vi "S4GUI.vi"(7 "Tab ObsEng":enum32{"Obs", "CCD modes", "Eng"}(tab)) -> ()   [LabVIEW 2018] (continued)
                      tunnel: [cluster{u32, u32}[] [{9868950, 9868950}, {9868950, 9868950}] ("Colors [4]") cluster{u32, u32}[] [{9868950, 9868950}, {9868950, 9868950}] ("Colors [4]") cluster{u32, u32}[] [{16318208, 16318208}, {16318208, 16318208}] ("Colors [4]") cluster{u32, u32}[] [{6618880, 6618880}, {6618880, 6618880}] ("Colors [4]") cluster{u32, u32}[] [{16318208, 16318208}, {16318208, 16318208}] ("Colors [4]")] -> w472
                      tunnel: [FALSE ("WPROT Status") FALSE ("WPROT Status") TRUE ("WPROT Status") FALSE ("WPROT Status") TRUE ("WPROT Status")] -> w471
                      frame Default {
                      }
                      frame 0 {
                      }
                      frame 1 {
                      }
                      frame 2 {
                      }
                      frame 3 {
                      }
                    }
                    "WPROT Status" <- w471
                    n230 = property on="WPROT Status" class="Bool (strict)"("Colors [4]"=w472) -> ()  [unwired: 2 in, 2 out]
                  }
                  frame #2 {
                    # "CALW"
                    n231 = Unbundle By Name(w492) -> ("CALW State"=w491:i32)
                    n232 = Unbundle By Name(w490) -> ("CALW posname"=w489:string)
                    n233 = local read "CALW Status"() -> (w485:bool)
                    n234 = case shown="3" w491 {
                      tunnel: [cluster{u32, u32}[] [{9868950, 9868950}, {9868950, 9868950}] ("Colors [4]") cluster{u32, u32}[] [{9868950, 9868950}, {9868950, 9868950}] ("Colors [4]") cluster{u32, u32}[] [{16318208, 16318208}, {16318208, 16318208}] ("Colors [4]") cluster{u32, u32}[] [{6618880, 6618880}, {6618880, 6618880}] ("Colors [4]") w512] -> w486
                      tunnel: [FALSE ("WPROT Status") FALSE ("WPROT Status") TRUE ("WPROT Status") FALSE ("WPROT Status") w514] -> w488
                      tunnel: w489 -> [_ _ _ w503 _]
                      tunnel: ["" "" "" w502 ""] -> w487
                      tunnel: w485 -> [_ _ _ _ w513]
                      frame Default {
                      }
                      frame 0 {
                      }
                      frame 1 {
                      }
                      frame 2 {
                        n235 = case shown="\"SHUTTER\"" w503 {
                          tunnel: ["" "DEPOL" "POL" "OFF" "PIN" "SHT"] -> w502
                          frame Default {
                          }
                          frame "DEPOLARIZER" {
                          }
                          frame "POLARIZER" {
                          }
                          frame "OFF" {
                          }
                          frame "PINHOLE" {
                          }
                          frame "SHUTTER" {
                          }
                        }
                      }
                      frame 3 {
                        n236 = case shown="False" w513 {
                          tunnel: [cluster{u32, u32}[] [{7563008, 7563008}, {7563008, 7563008}] ("Colors [4]") cluster{u32, u32}[] [{16318208, 16318208}, {16318208, 16318208}] ("Colors [4]")] -> w512
                          frame False {
                          }
                          frame True {
                          }
                        }
                        n237 = Not(x=w513) -> (.not. x?=w514:bool)
                      }
                    }
                    "CALW Status" <- w488
                    "PCS" <- w488
                    n238 = property on="CALW Status" class="Bool (strict)"("Colors [4]"=w486) -> ()  [unwired: 2 in, 2 out]
                    n239 = property on="PCS" class="Bool (strict)"("Colors [4]"=w486, "BoolText.Text"=w487) -> ()  [unwired: 2 in, 2 out]
                  }
                  frame #3 {
                    # "ASEL"
                    n240 = Unbundle By Name(w526) -> ("ASEL State"=w525:i32)
                    n241 = Unbundle By Name(w522) -> ("ASEL posname"=w519:string)
                    n242 = local read "ASEL Status"() -> (w520:bool)
                    n243 = case shown="Default" w519 {
                      selector: w519 -> [w527 _ _]
                      tunnel: [w527 "OFF" ("y") "ON" ("y")] -> w518
                      frame Default {
                      }
                      frame "OFF" {
                      }
                      frame "ON" {
                      }
                    }
                    n244 = case shown="3" w525 {
                      tunnel: [cluster{u32, u32}[] [{9868950, 9868950}, {9868950, 9868950}] ("Colors [4]") cluster{u32, u32}[] [{9868950, 9868950}, {9868950, 9868950}] ("Colors [4]") cluster{u32, u32}[] [{16318208, 16318208}, {16318208, 16318208}] ("Colors [4]") cluster{u32, u32}[] [{6618880, 6618880}, {6618880, 6618880}] ("Colors [4]") w545] -> w523
                      tunnel: [FALSE ("WPROT Status") FALSE ("WPROT Status") TRUE FALSE ("WPROT Status") w544] -> w524
                      tunnel: w518 -> [_ _ _ w540 _]
                      tunnel: ["" ("y") "" ("y") "" ("y") w540 "" ("y")] -> w521
                      tunnel: w520 -> [_ _ _ _ w542]
                      frame Default {
                      }
                      frame 0 {
                      }
                      frame 1 {
                      }
                      frame 2 {
                      }
                      frame 3 {
                        n245 = case shown="True" w542 {
                          tunnel: [cluster{u32, u32}[] [{7563008, 7563008}, {7563008, 7563008}] ("Colors [4]") cluster{u32, u32}[] [{16318208, 16318208}, {16318208, 16318208}] ("Colors [4]")] -> w545
                          frame False {
                          }
                          frame True {
                          }
                        }
                        n246 = Not(x=w542) -> (.not. x?=w544:bool)
                      }
                    }
                    "ASEL Status" <- w524
                    "Analyzer" <- w524
                    n247 = property on="Analyzer" class="Bool (strict)"("Colors [4]"=w523, "BoolText.Text"=w521) -> ()  [unwired: 2 in, 2 out]
                    n248 = property on="ASEL Status" class="Bool (strict)"("Colors [4]"=w523) -> ()  [unwired: 2 in, 2 out]
                  }
                  frame #4 {
                    # "GMIR"
                    n249 = Unbundle By Name(w551) -> ("GMIR State"=w550:i32)
                    n250 = case shown="0" w550 {
                      tunnel: [cluster{u32, u32}[] [{9868950, 9868950}, {9868950, 9868950}] ("Colors [4]") cluster{u32, u32}[] [{9868950, 9868950}, {9868950, 9868950}] ("Colors [4]") cluster{u32, u32}[] [{16318208, 16318208}, {16318208, 16318208}] ("Colors [4]") cluster{u32, u32}[] [{6618880, 6618880}, {6618880, 6618880}] ("Colors [4]") cluster{u32, u32}[] [{16318208, 16318208}, {16318208, 16318208}] ("Colors [4]")] -> w549
                      tunnel: [FALSE ("WPROT Status") FALSE ("WPROT Status") TRUE ("WPROT Status") FALSE ("WPROT Status") TRUE ("WPROT Status")] -> w548
                      frame Default {
                      }
                      frame 0 {
                      }
                      frame 1 {
                      }
                      frame 2 {
                      }
                      frame 3 {
                      }
                    }
                    "GMIR Status" <- w548
                    n251 = property on="GMIR Status" class="Bool (strict)"("Colors [4]"=w549) -> ()  [unwired: 2 in, 2 out]
                  }
                  frame #5 {
                    # "GFOC"
                    n252 = Unbundle By Name(w565) -> ("GFOC State"=w564:i32)
                    n253 = case shown="2" w564 {
                      tunnel: [cluster{u32, u32}[] [{9868950, 9868950}, {9868950, 9868950}] ("Colors [4]") cluster{u32, u32}[] [{9868950, 9868950}, {9868950, 9868950}] ("Colors [4]") cluster{u32, u32}[] [{16318208, 16318208}, {16318208, 16318208}] ("Colors [4]") cluster{u32, u32}[] [{6618880, 6618880}, {6618880, 6618880}] ("Colors [4]") cluster{u32, u32}[] [{16318208, 16318208}, {16318208, 16318208}] ("Colors [4]")] -> w563
                      tunnel: [FALSE ("WPROT Status") FALSE ("WPROT Status") TRUE ("WPROT Status") FALSE ("WPROT Status") TRUE ("WPROT Status")] -> w562
                      frame Default {
                      }
                      frame 0 {
                      }
                      frame 1 {
                      }
                      frame 2 {
                      }
                      frame 3 {
                      }
                    }
                    "GFOC Status" <- w562
                    n254 = property on="GFOC Status" class="Bool (strict)"("Colors [4]"=w563) -> ()  [unwired: 2 in, 2 out]
                  }
                }
              }
              frame #7 {
                n255 = Unbundle By Name(w578) -> ("Instrument Pos Names"=w577:T20)
                n256 = stacked-sequence {
                  tunnel: w577 -> [w580 w597 w622 w648]
                  tunnel: [_ _ _ w649] -> w576
                  frame #0 {
                    n257 = Unbundle By Name(w580) -> ("WPSEL posname"=w579:string)
                    n258 = case shown="\"L/2\", \"L/4\", \"OFF\"" w579 {
                      selector: w579 -> [_ w581]
                      frame "False", Default {
                      }
                      frame "L/2", "L/4", "OFF" {
                        n259 = First Call?() -> (First Call?: T/F=w582:bool)
                        n260 = case shown="True" w582 {
                          tunnel: w581 -> [_ w583]
                          frame False {
                          }
                          frame True {
                            n261 = case shown="\"L/2\"" w583 {
                              frame "False", Default {
                              }
                              frame "L/2" {
                                w584 = u16 1 items=["OFF", "Lambda/2", "Lambda/4"] ("Lambda Selector")
                                n262 = property on="Lambda Selector" class="Ring (strict)"(error in=errorcluster {"status"=FALSE, "code"=0, "source"=""} ("error in (no error)"), "Value"=w584) -> (error out=w586:errorcluster)  [unwired: 1 in, 1 out]
                                n263 = property on="Lambda Selector" class="Ring (strict)"(error in=w586, "RingText.Text"="Lambda/2" ("Boolean Text.Text")) -> ()  [unwired: 1 in, 2 out]
                              }
                              frame "L/4" {
                                w588 = u16 2 items=["OFF", "Lambda/2", "Lambda/4"] ("Lambda Selector")
                                n264 = property on="Lambda Selector" class="Ring (strict)"(error in=errorcluster {"status"=FALSE, "code"=0, "source"=""} ("error in (no error)"), "Value"=w588) -> (error out=w590:errorcluster)  [unwired: 1 in, 1 out]
                                n265 = property on="Lambda Selector" class="Ring (strict)"(error in=w590, "RingText.Text"="Lambda/4" ("Boolean Text.Text")) -> ()  [unwired: 1 in, 2 out]
                              }
                              frame "OFF" {
                                w592 = u16 0 items=["OFF", "Lambda/2", "Lambda/4"] ("Lambda Selector")
                                n266 = property on="Lambda Selector" class="Ring (strict)"(error in=errorcluster {"status"=FALSE, "code"=0, "source"=""} ("error in (no error)"), "Value"=w592) -> (error out=w594:errorcluster)  [unwired: 1 in, 1 out]
                                n267 = property on="Lambda Selector" class="Ring (strict)"(error in=w594, "RingText.Text"="OFF" ("Boolean Text.Text")) -> ()  [unwired: 1 in, 2 out]
                              }
                            }
                          }
                        }
                      }
                    }
                  }
                  frame #1 {
                    n268 = Unbundle By Name(w597) -> ("CALW posname"=w596:string)
                    n269 = case shown="\"DEPOLARIZER\", \"OFF\", \"PINHOLE\", \"POLARIZER\", \"SHUTTER\"" w596 {
                      selector: w596 -> [_ w598]
                      frame "False", Default {
                      }
                      frame "DEPOLARIZER", "OFF", "PINHOLE", "POLARIZER", "SHUTTER" {
                        n270 = First Call?() -> (First Call?: T/F=w599:bool)
                        n271 = case shown="True" w599 {
                          tunnel: w598 -> [_ w600]
                          frame False {
                          }
                          frame True {
                            n272 = case shown="\"OFF\"" w600 {
                              frame "False", Default {
                              }
                              frame "POLARIZER" {
                                w601 = u16 1 items=["OFF", "POLARIZER", "PINHOLE", "SHUTTER", "DEPOLARIZER"] ("Calibrator Selector")
                                n273 = property on="Calibrator Selector" class="Ring (strict)"(error in=errorcluster {"status"=FALSE, "code"=0, "source"=""} ("error in (no error)"), "Value"=w601) -> (error out=w603:errorcluster)  [unwired: 1 in, 1 out]
                                n274 = property on="Calibrator Selector" class="Ring (strict)"(error in=w603, "RingText.Text"="POLARIZER" ("Boolean Text.Text")) -> ()  [unwired: 1 in, 2 out]
                              }
                              frame "DEPOLARIZER" {
                                w605 = u16 4 items=["OFF", "POLARIZER", "PINHOLE", "SHUTTER", "DEPOLARIZER"] ("Calibrator Selector")
                                n275 = property on="Calibrator Selector" class="Ring (strict)"(error in=errorcluster {"status"=FALSE, "code"=0, "source"=""} ("error in (no error)"), "Value"=w605) -> (error out=w607:errorcluster)  [unwired: 1 in, 1 out]
                                n276 = property on="Calibrator Selector" class="Ring (strict)"(error in=w607, "RingText.Text"="DEPOLARIZER" ("Boolean Text.Text")) -> ()  [unwired: 1 in, 2 out]
                              }
                              frame "PINHOLE" {
                                w609 = u16 2 items=["OFF", "POLARIZER", "PINHOLE", "SHUTTER", "DEPOLARIZER"] ("Calibrator Selector")
                                n277 = property on="Calibrator Selector" class="Ring (strict)"(error in=errorcluster {"status"=FALSE, "code"=0, "source"=""} ("error in (no error)"), "Value"=w609) -> (error out=w611:errorcluster)  [unwired: 1 in, 1 out]
                                n278 = property on="Calibrator Selector" class="Ring (strict)"(error in=w611, "RingText.Text"="PINHOLE" ("Boolean Text.Text")) -> ()  [unwired: 1 in, 2 out]
                              }
                              frame "SHUTTER" {
                                w613 = u16 3 items=["OFF", "POLARIZER", "PINHOLE", "SHUTTER", "DEPOLARIZER"] ("Calibrator Selector")
                                n279 = property on="Calibrator Selector" class="Ring (strict)"(error in=errorcluster {"status"=FALSE, "code"=0, "source"=""} ("error in (no error)"), "Value"=w613) -> (error out=w615:errorcluster)  [unwired: 1 in, 1 out]
                                n280 = property on="Calibrator Selector" class="Ring (strict)"(error in=w615, "RingText.Text"="SHUTTER" ("Boolean Text.Text")) -> ()  [unwired: 1 in, 2 out]
                              }
                              frame "OFF" {
                                w617 = u16 0 items=["OFF", "POLARIZER", "PINHOLE", "SHUTTER", "DEPOLARIZER"] ("Calibrator Selector")
                                n281 = property on="Calibrator Selector" class="Ring (strict)"(error in=errorcluster {"status"=FALSE, "code"=0, "source"=""} ("error in (no error)"), "Value"=w617) -> (error out=w619:errorcluster)  [unwired: 1 in, 1 out]
                                n282 = property on="Calibrator Selector" class="Ring (strict)"(error in=w619, "RingText.Text"="OFF" ("Boolean Text.Text")) -> ()  [unwired: 1 in, 2 out]
                              }
                            }
                          }
                        }
                      }
                    }
                  }
                  frame #2 {
                    n283 = Unbundle By Name(w622) -> ("WPROT posname"=w621:string)
                    "Name" <- w621
                    n284 = stacked-sequence {
                      tunnel: w621 -> [_ w624]
                      frame #0 {
                        w623 = FALSE
                        "ledP0" <- w623
                        "ledP1" <- w623
                        "ledP2" <- w623
                        "ledP3" <- w623
                        "ledP4" <- w623
                        "ledP5" <- w623
                        "ledP6" <- w623
                        "ledP7" <- w623
                        "ledP8" <- w623
                        "ledP9" <- w623
                        "ledP10" <- w623
                        "ledP11" <- w623
                        "ledP12" <- w623
                        "ledP13" <- w623
                        "ledP14" <- w623
                        "ledP15" <- w623
                      }
                      frame #1 {
                        n285 = case shown="\"WP3\"" w624 {
                          frame Default {
                          }
                          frame "WP1" {
                            n286 = local write "ledP0"(TRUE ("ledP0")) -> ()
                          }
                          frame "WP2" {
                            n287 = local write "ledP1"(TRUE ("ledP0")) -> ()
                          }
                          frame "WP3" {
                            n288 = local write "ledP2"(TRUE ("ledP0")) -> ()
                          }
                          frame "WP4" {
                            n289 = local write "ledP3"(TRUE ("ledP0")) -> ()
                          }
                          frame "WP5" {
                            n290 = local write "ledP4"(TRUE ("ledP0")) -> ()
                          }
                          frame "WP6" {
                            n291 = local write "ledP5"(TRUE ("ledP0")) -> ()
                          }
                          frame "WP7" {
                            n292 = local write "ledP6"(TRUE ("ledP0")) -> ()
                          }
                          frame "WP8" {
                            n293 = local write "ledP7"(TRUE ("ledP0")) -> ()
                          }
                          frame "WP9" {
                            n294 = local write "ledP8"(TRUE ("ledP0")) -> ()
                          }
                          frame "WP10" {
                            n295 = local write "ledP9"(TRUE ("ledP0")) -> ()
                          }
                          frame "WP11" {
                            n296 = local write "ledP10"(TRUE ("ledP0")) -> ()
                          }
                          frame "WP12" {
                            n297 = local write "ledP11"(TRUE ("ledP0")) -> ()
                          }
                          frame "WP13" {
                            n298 = local write "ledP12"(TRUE ("ledP0")) -> ()
                          }
                          frame "WP14" {
                            n299 = local write "ledP13"(TRUE ("ledP0")) -> ()
                          }
                          frame "WP15" {
                            n300 = local write "ledP14"(TRUE ("ledP0")) -> ()
                          }
                          frame "WP16" {
                            n301 = local write "ledP15"(TRUE ("ledP0")) -> ()
                          }
                        }
                      }
                    }
                  }
                  frame #3 {
                    w652 = "OFF" ("Boolean Text.Text")
                    # "Polarimetria:   ASEL = ON  &   (WPSEL =L/2 or L/4)\n\nFotometria:    ASEL=OFF & WPSEL = OFF & CALW = OFF"
                    n302 = Unbundle By Name(w648) -> ("ASEL posname"=w643:string, "WPSEL posname"=w645:string, "CALW posname"=w644:string)
                    n303 = Unbundle By Name(w648) -> ("WPSEL posname"=w655:string, "CALW posname"=w656:string, "ASEL posname"=w650:string)
                    n304 = Equal?(x=w643, y="ON" ("Boolean Text.Text")) -> (x = y?=w646:bool)
                    n305 = case shown="True" w646 {
                      tunnel: w645 -> [w665 w674]
                      tunnel: w644 -> [w664 w668]
                      tunnel: w643 -> [w661 _]
                      tunnel: [FALSE ("Polarimetric Mode") w669] -> w642
                      tunnel: [w657 FALSE ("Photometric Mode")] -> w641
                      frame False {
                        w660 = "OFF" ("Boolean Text.Text")
                        n306 = Equal?(x=w661, y=w660) -> (x = y?=w659:bool)
                        n307 = Equal?(x=w664, y=w660) -> (x = y?=w662:bool)
                        n308 = Equal?(x=w665, y=w660) -> (x = y?=w663:bool)
                        n309 = Compound Arithmetic op=AND(w659, w663, w662) -> (w657:bool)
                      }
                      frame True {
                        n310 = Equal?(x="L/2" ("Boolean Text.Text"), y=w674) -> (x = y?=w675:bool)
                        n311 = Equal?(x="L/4" ("Boolean Text.Text"), y=w674) -> (x = y?=w672:bool)
                        n312 = Not Equal?(x="SHUTTER", y=w668) -> (x != y?=w666:bool)
                        n313 = Or(x=w675, y=w672) -> (x .or. y?=w670:bool)
                        n314 = And(x=w670, y=w666) -> (x .and. y?=w669:bool)
                      }
                    }
                    "Polarimetric Mode" <- w642
                    "Photometric Mode" <- w641
                    n315 = Equal?(x=w652, y=w655) -> (x = y?=w653:bool)
                    n316 = Equal?(x=w652, y=w656) -> (x = y?=w654:bool)
                    n317 = Equal?(x=w652, y=w650) -> (x = y?=w651:bool)
                    n318 = Compound Arithmetic op=AND(w653, w654, w651) -> (invert w649:bool)
                  }
                }
              }
              frame #8 {
                n319 = Unbundle By Name(w681) -> ("ChannelA_Status"=w680:T21, "ChannelB_Status"=w679:T21, "ChannelC_Status"=w677:T21, "ChannelD_Status"=w678:T21)
                n320 = stacked-sequence {
                  tunnel: w680 -> [w769 w825 w877 w954 _ _ _]
                  tunnel: w679 -> [w768 w823 w876 _ w975 _ _]
                  tunnel: w678 -> [w766 w820 w874 _ _ _ w1017]
                  tunnel: w677 -> [w767 w821 w875 _ _ w996 _]
                  frame #0 {
                    n321 = Unbundle By Name(w766) -> ("connection"=w746:bool, "FT"=w727:bool, "Current exp"=w704:dbl, "Cooler ON/OFF"=w760:i16, "Currently temperature"=w757:i16, "Temperature Status"=w754:string, "target  temp"=w689:i16)
                    "Exposure Time ch4" <- w704
                    n322 = Unbundle By Name(w768) -> ("connection"=w748:bool, "FT"=w731:bool, "Current exp"=w715:dbl, "Cooler ON/OFF"=w762:i16, "Currently temperature"=w759:i16, "Temperature Status"=w756:string, "target  temp"=w693:i16)
                    "Exposure Time ch2" <- w715
                    n323 = Unbundle By Name(w769) -> ("connection"=w749:bool, "FT"=w732:bool, "Current exp"=w724:dbl, "Cooler ON/OFF"=w765:i16, "Currently temperature"=w763:i16, "Temperature Status"=w764:string, "target  temp"=w701:i16)
                    "Exposure Time ch1" <- w724
                    n324 = Unbundle By Name(w767) -> ("connection"=w747:bool, "FT"=w729:bool, "Current exp"=w705:dbl, "Cooler ON/OFF"=w761:i16, "Currently temperature"=w758:i16, "Temperature Status"=w755:string, "target  temp"=w690:i16)
                    "Exposure Time ch3" <- w705
                    n325 = Number To Decimal String(number=w689) -> (decimal integer string=→"Target Temp 4":string)  [unwired: 1 in]
                    n326 = Number To Decimal String(number=w690) -> (decimal integer string=→"Target Temp 3":string)  [unwired: 1 in]
                    n327 = Number To Decimal String(number=w693) -> (decimal integer string=→"Target Temp 2":string)  [unwired: 1 in]
                    n328 = Not Equal To 0?(x=w760) -> (x != 0?=w751:bool)
                    n329 = First Call?() -> (First Call?: T/F=w743:bool)
                    n330 = First Call?() -> (First Call?: T/F=w745:bool)
                    n331 = First Call?() -> (First Call?: T/F=w742:bool)
                    n332 = Not Equal To 0?(x=w761) -> (x != 0?=w750:bool)
                    n333 = First Call?() -> (First Call?: T/F=w744:bool)
                    n334 = Number To Decimal String(number=w701) -> (decimal integer string=→"Target Temp 1":string)  [unwired: 1 in]
                    n335 = Number To Fractional String(use system decimal point (T)=FALSE, number=w724, precision (6)=i16 2) -> (F-format string=w721:string)  [unwired: 1 in]
                    n336 = case shown="True" w743 {
                      tunnel: w690 -> [_ w771]
                      frame False {
                      }
                      frame True {
                        n337 = property on="Target Temp 3" class="DigNum (strict)"("Value"=w771) -> ()  [unwired: 2 in, 2 out]
                      }
                    }
                    n338 = case shown="True" w745 {
                      tunnel: w701 -> [_ w773]
                      frame False {
                      }
                      frame True {
                        n339 = property on="Target Temp 1" class="DigNum (strict)"("Value"=w773) -> ()  [unwired: 2 in, 2 out]
                      }
                    }
                    n340 = Number To Fractional String(use system decimal point (T)=FALSE, number=w715, precision (6)=i16 2) -> (F-format string=w716:string)  [unwired: 1 in]
                    n341 = case shown="True" w742 {
                      tunnel: w689 -> [_ w770]
                      frame False {
                      }
                      frame True {
                        n342 = property on="Target Temp 4" class="DigNum (strict)"("Value"=w770) -> ()  [unwired: 2 in, 2 out]
                      }
                    }
                    n343 = Concatenate Strings("Exposure Time ", w721) -> (w720:string)
                    n344 = Number To Fractional String(use system decimal point (T)=FALSE, number=w705, precision (6)=i16 2) -> (F-format string=w706:string)  [unwired: 1 in]
                    n345 = Number To Fractional String(use system decimal point (T)=FALSE, number=w704, precision (6)=i16 2) -> (F-format string=w710:string)  [unwired: 1 in]
                    n346 = Concatenate Strings("Exposure Time ", w716) -> (w714:string)
                    n347 = case shown="True" w744 {
                      tunnel: w693 -> [_ w772]
                      frame False {
                      }
                      frame True {
                        n348 = property on="Target Temp 2" class="DigNum (strict)"("Value"=w772) -> ()  [unwired: 2 in, 2 out]
                      }
                    }
                    n349 = Concatenate Strings("Exposure Time ", w706) -> (w702:string)
                    n350 = Concatenate Strings("Exposure Time ", w710) -> (w703:string)
                    n351 = property on="Exposure Time ch1" class="Slide (strict)"("Caption.Text"=w720) -> ()  [unwired: 2 in, 2 out]
                    n352 = property on="Exposure Time ch2" class="Slide (strict)"("Caption.Text"=w714) -> ()  [unwired: 2 in, 2 out]
                    n353 = property on="Exposure Time ch3" class="Slide (strict)"("Caption.Text"=w702) -> ()  [unwired: 2 in, 2 out]
                    n354 = property on="Exposure Time ch4" class="Slide (strict)"("Caption.Text"=w703) -> ()  [unwired: 2 in, 2 out]
                    n355 = Not Equal To 0?(x=w765) -> (x != 0?=w752:bool)
                    n356 = Not Equal To 0?(x=w762) -> (x != 0?=w753:bool)
                    n357 = case shown="False" w749 {
                      tunnel: w764 -> [_ w803]
                      tunnel: w763 -> [_ w804]
                      tunnel: w752 -> [_ w805]
                      tunnel: [FALSE w805] -> w741
                      tunnel: [i16 0 ("Currently temperature") w804] -> w698
                      tunnel: ["" ("Temperature Status") w803] -> w740
                      tunnel: [FALSE w802] -> w733
                      tunnel: w732 -> [_ w802]
                      frame False {
                      }
                      frame True {
                      }
                    }
                    "Cooler status 1" <- w741
                    "Curr Temp 1" <- w698
                    "Temp Status 1" <- w740
                    "Panel Temp" <- w698
                    "Panel cooler 1" <- w741
                    "FT1" <- w733
                    n358 = case shown="False" w748 {
                      tunnel: w759 -> [_ w796]
                      tunnel: w756 -> [_ w795]
                      tunnel: w753 -> [_ w797]
                      tunnel: [FALSE w797] -> w739
                      tunnel: [i16 0 ("Currently temperature") w796] -> w694
                      tunnel: ["" ("Temperature Status") w795] -> w738
                      tunnel: w731 -> [_ w794]
                      tunnel: [FALSE ("FT") w794] -> w730
                      frame False {
                      }
                      frame True {
                      }
                    }
                    "Panel Temp 2" <- w694
                    "Curr Temp 2" <- w694
                    "Cooler status 2" <- w739
                    "Panel cooler 2" <- w739
                    "Temp Status 2" <- w738
                    "FT2" <- w730
                    n359 = case shown="True" w746 {
                      tunnel: w757 -> [_ w780]
                      tunnel: w754 -> [_ w779]
                      tunnel: w751 -> [_ w781]
                      tunnel: [FALSE w781] -> w735
                      tunnel: [i16 0 ("Currently temperature") w780] -> w682
                      tunnel: ["" ("Temperature Status") w779] -> w734
                      tunnel: w727 -> [_ w778]
                      tunnel: [FALSE ("FT") w778] -> w726
                      frame False {
                      }
                      frame True {
                      }
                    }
                    "Cooler status 4" <- w735
                    "Panel Temp 4" <- w682
                    "Curr Temp 4" <- w682
                    "Temp Status 4" <- w734
                    "Panel cooler 4" <- w735
                    "FT4" <- w726
                    n360 = case shown="True" w747 {
                      tunnel: w758 -> [_ w788]
                      tunnel: w755 -> [_ w787]
                      tunnel: w750 -> [_ w789]
                      tunnel: [FALSE w789] -> w737
                      tunnel: [i16 0 ("Currently temperature") w788] -> w683
                      tunnel: ["" ("Temperature Status") w787] -> w736
                      tunnel: w729 -> [_ w786]
                      tunnel: [FALSE ("FT") w786] -> w728
                      frame False {
                      }
                      frame True {
                      }
                    }
                    "Cooler status 3" <- w737
                    "Panel Temp 3" <- w683
                    "Curr Temp 3" <- w683
                    "Temp Status 3" <- w736
                    "Panel cooler 3" <- w737
                    "FT3" <- w728
                    n361 = Number To Decimal String(number=w694) -> (decimal integer string=w695:string)  [unwired: 1 in]
                    n362 = Number To Decimal String(number=w698) -> (decimal integer string=w699:string)  [unwired: 1 in]
                    n363 = property on="Panel cooler 2" class="Bool (strict)"("BoolText.Text"=w695, "BoolText.Justify"=enum16{"Left", "Center", "Right"}."Right" ("Boolean Text.Justification")) -> ()  [unwired: 2 in, 2 out]
                    n364 = property on="Panel cooler 1" class="Bool (strict)"("BoolText.Text"=w699, "BoolText.Justify"=enum16{"Left", "Center", "Right"}."Right" ("Boolean Text.Justification")) -> ()  [unwired: 2 in, 2 out]
                    n365 = Number To Decimal String(number=w683) -> (decimal integer string=w687:string)  [unwired: 1 in]
                    n366 = Number To Decimal String(number=w682) -> (decimal integer string=w684:string)  [unwired: 1 in]
                    n367 = property on="Panel cooler 3" class="Bool (strict)"("BoolText.Text"=w687, "BoolText.Justify"=enum16{"Left", "Center", "Right"}."Right" ("Boolean Text.Justification")) -> ()  [unwired: 2 in, 2 out]
                    n368 = property on="Panel cooler 4" class="Bool (strict)"("BoolText.Text"=w684, "BoolText.Justify"=enum16{"Left", "Center", "Right"}."Right" ("Boolean Text.Justification")) -> ()  [unwired: 2 in, 2 out]
                  }
                  frame #1 {
                    n369 = Unbundle By Name(w820) -> ("LastFileImage"=→"Last Image ch4":string, "Temperature Status"=w808:string)
                    n370 = Unbundle By Name(w821) -> ("LastFileImage"=→"Last Image ch3":string, "Temperature Status"=w809:string)
                    n371 = Unbundle By Name(w823) -> ("LastFileImage"=→"Last Image ch2":string, "Temperature Status"=w812:string)
                    n372 = Unbundle By Name(w825) -> ("LastFileImage"=→"Last Image ch1":string, "Temperature Status"=w817:string)
                    n373 = case shown="\"TEMPERATURE_NOT_REACHED\"" w817 {
                      tunnel: [cluster{u32, u32}[] [{6124107, 6124107}, {6124107, 6124107}] ("Colors [4]") cluster{u32, u32}[] [{6618880, 6618880}, {6618880, 6618880}] ("Colors [4]") cluster{u32, u32}[] [{16318208, 16318208}, {16318208, 16318208}] ("Colors [4]") cluster{u32, u32}[] [{8554752, 8554752}, {8554752, 8554752}] ("Colors [4]")] -> w816
                      tunnel: [FALSE FALSE FALSE TRUE] -> w815
                      frame Default {
                      }
                      frame "TEMPERATURE_STABILIZED" {
                      }
                      frame "TEMPERATURE_NOT_STABILIZED" {
                      }
                      frame "TEMPERATURE_NOT_REACHED" {
                      }
                    }
                    n374 = case shown="\"TEMPERATURE_NOT_REACHED\"" w812 {
                      tunnel: [cluster{u32, u32}[] [{6124107, 6124107}, {6124107, 6124107}] ("Colors [4]") cluster{u32, u32}[] [{6618880, 6618880}, {6618880, 6618880}] ("Colors [4]") cluster{u32, u32}[] [{16318208, 16318208}, {16318208, 16318208}] ("Colors [4]") cluster{u32, u32}[] [{8554752, 8554752}, {8554752, 8554752}] ("Colors [4]")] -> w814
                      tunnel: [FALSE FALSE FALSE TRUE] -> w813
                      frame Default {
                      }
                      frame "TEMPERATURE_STABILIZED" {
                      }
                      frame "TEMPERATURE_NOT_STABILIZED" {
                      }
                      frame "TEMPERATURE_NOT_REACHED" {
                      }
                    }
                    n375 = case shown="\"TEMPERATURE_NOT_REACHED\"" w809 {
                      tunnel: [cluster{u32, u32}[] [{6124107, 6124107}, {6124107, 6124107}] ("Colors [4]") cluster{u32, u32}[] [{6618880, 6618880}, {6618880, 6618880}] ("Colors [4]") cluster{u32, u32}[] [{16318208, 16318208}, {16318208, 16318208}] ("Colors [4]") cluster{u32, u32}[] [{8554752, 8554752}, {8554752, 8554752}] ("Colors [4]")] -> w811
                      tunnel: [FALSE FALSE FALSE TRUE] -> w810
                      frame Default {
                      }
                      frame "TEMPERATURE_STABILIZED" {
                      }
                      frame "TEMPERATURE_NOT_STABILIZED" {
                      }
                      frame "TEMPERATURE_NOT_REACHED" {
                      }
                    }
                    n376 = case shown="\"TEMPERATURE_NOT_REACHED\"" w808 {
                      tunnel: [cluster{u32, u32}[] [{6124107, 6124107}, {6124107, 6124107}] ("Colors [4]") cluster{u32, u32}[] [{6618880, 6618880}, {6618880, 6618880}] ("Colors [4]") cluster{u32, u32}[] [{16318208, 16318208}, {16318208, 16318208}] ("Colors [4]") cluster{u32, u32}[] [{8554752, 8554752}, {8554752, 8554752}] ("Colors [4]")] -> w807
                      tunnel: [FALSE FALSE FALSE TRUE] -> w806
                      frame Default {
                      }
                      frame "TEMPERATURE_STABILIZED" {
                      }
                      frame "TEMPERATURE_NOT_STABILIZED" {
                      }
                      frame "TEMPERATURE_NOT_REACHED" {
                      }
                    }
                    n377 = property on="Cooler status 1" class="Bool (strict)"("Colors [4]"=w816, "Blinking"=w815) -> ()  [unwired: 2 in, 2 out]
                    n378 = property on="Panel cooler 1" class="Bool (strict)"("Colors [4]"=w816, "Blinking"=w815) -> ()  [unwired: 2 in, 2 out]
                    n379 = property on="Cooler status 4" class="Bool (strict)"("Colors [4]"=w807, "Blinking"=w806) -> ()  [unwired: 2 in, 2 out]
                    n380 = property on="Cooler status 3" class="Bool (strict)"("Colors [4]"=w811, "Blinking"=w810) -> ()  [unwired: 2 in, 2 out]
                    n381 = property on="Panel cooler 4" class="Bool (strict)"("Colors [4]"=w807, "Blinking"=w806) -> ()  [unwired: 2 in, 2 out]
                    n382 = property on="Cooler status 2" class="Bool (strict)"("Colors [4]"=w814, "Blinking"=w813) -> ()  [unwired: 2 in, 2 out]
                    n383 = property on="Panel cooler 3" class="Bool (strict)"("Colors [4]"=w811, "Blinking"=w810) -> ()  [unwired: 2 in, 2 out]
                    n384 = property on="Panel cooler 2" class="Bool (strict)"("Colors [4]"=w814, "Blinking"=w813) -> ()  [unwired: 2 in, 2 out]
                  }
                  frame #2 {
                    n385 = Unbundle By Name(w876) -> ("CamStatus"=w869:string, "connection"=w868:bool)
                    n386 = Unbundle By Name(w875) -> ("CamStatus"=w865:string, "connection"=w864:bool)
                    n387 = Unbundle By Name(w874) -> ("CamStatus"=w861:string, "connection"=w860:bool)
                    n388 = Unbundle By Name(w877) -> ("CamStatus"=w873:string, "connection"=w871:bool)
                    n389 = case shown="True" w868 {
                      tunnel: w869 -> [_ w908]
                      tunnel: [u32 16739417 w909] -> w866
                      tunnel: ["" ("CamStatus") w908] -> w867
                      frame False {
                      }
                      frame True {
                        n390 = property on="Acq status string ch2" class="Str"() -> ("Text.BGColor"=w910:u32)  [unwired: 2 in, 2 out]
                        n391 = case shown="\"\"" w908 {
                          tunnel: [u32 16688641 w915 u32 13882323 u32 13882323] -> w909
                          tunnel: w910 -> [_ w914 _ _]
                          frame Default {
                            # "WAITING_EXPOSE_COMMAND"
                          }
                          frame "ACTIVE" {
                            n392 = Equal?(x=w914, y=u32 16776002) -> (x = y?=w913:bool)
                            n393 = case shown="False" w913 {
                              tunnel: [u32 16776002 u32 16449369] -> w915
                              frame False {
                              }
                              frame True {
                              }
                            }
                          }
                          frame "IDLE" {
                          }
                          frame "" {
                            # "sem resposta do ACS"
                          }
                        }
                      }
                    }
                    "Acq status string ch2" <- w867
                    n394 = case shown="True" w860 {
                      tunnel: w861 -> [_ w880]
                      tunnel: [u32 16739417 w881] -> w858
                      tunnel: ["" ("CamStatus") w880] -> w859
                      frame False {
                      }
                      frame True {
                        n395 = property on="Acq status string ch4" class="Str"() -> ("Text.BGColor"=w882:u32)  [unwired: 2 in, 2 out]
                        n396 = case shown="\"IDLE\"" w880 {
                          tunnel: [u32 16688641 w887 u32 13882323 u32 13882323] -> w881
                          tunnel: w882 -> [_ w886 _ _]
                          frame Default {
                            # "WAITING_EXPOSE_COMMAND"
                          }
                          frame "ACTIVE" {
                            n397 = Equal?(x=w886, y=u32 16776002) -> (x = y?=w885:bool)
                            n398 = case shown="False" w885 {
                              tunnel: [u32 16776002 u32 16449369] -> w887
                              frame False {
                              }
                              frame True {
                              }
                            }
                          }
                          frame "IDLE" {
                          }
                          frame "" {
                            # "sem resposta do ACS"
                          }
                        }
                      }
                    }
                    "Acq status string ch4" <- w859
                    n399 = case shown="True" w864 {
                      tunnel: w865 -> [_ w894]
                      tunnel: [u32 16739417 w895] -> w862
                      tunnel: ["" ("CamStatus") w894] -> w863
                      frame False {
                      }
                      frame True {
                        n400 = property on="Acq status string ch3" class="Str"() -> ("Text.BGColor"=w896:u32)  [unwired: 2 in, 2 out]
                        n401 = case shown="\"\"" w894 {
                          tunnel: [u32 16688641 w901 u32 13882323 u32 13882323] -> w895
                          tunnel: w896 -> [_ w900 _ _]
                          frame Default {
                            # "WAITING_EXPOSE_COMMAND"
                          }
                          frame "ACTIVE" {
                            n402 = Equal?(x=w900, y=u32 16776002) -> (x = y?=w899:bool)
                            n403 = case shown="False" w899 {
                              tunnel: [u32 16776002 u32 16449369] -> w901
                              frame False {
                              }
                              frame True {
                              }
                            }
                          }
                          frame "IDLE" {
                          }
                          frame "" {
                            # "sem resposta do ACS"
                          }
                        }
                      }
                    }
                    "Acq status string ch3" <- w863
                    n404 = case shown="True" w871 {
                      tunnel: w873 -> [_ w922]
                      tunnel: [u32 16739417 w923] -> w872
                      tunnel: ["" ("CamStatus") w922] -> w870
                      frame False {
                      }
                      frame True {
                        n405 = property on="Acq status string ch1" class="Str"() -> ("Text.BGColor"=w924:u32)  [unwired: 2 in, 2 out]
                        n406 = case shown="\"\"" w922 {
                          tunnel: [u32 16688641 w929 u32 13882323 u32 13882323] -> w923
                          tunnel: w924 -> [_ w928 _ _]
                          frame Default {
                            # "WAITING_EXPOSE_COMMAND"
                          }
                          frame "ACTIVE" {
                            n407 = Equal?(x=w928, y=u32 16776002) -> (x = y?=w927:bool)
                            n408 = case shown="False" w927 {
                              tunnel: [u32 16776002 u32 16449369] -> w929
                              frame False {
                              }
                              frame True {
                              }
                            }
                          }
                          frame "IDLE" {
                          }
                          frame "" {
                            # "sem resposta do ACS"
                          }
                        }
                      }
                    }
                    "Acq status string ch1" <- w870
                    n409 = property on="Acq status string ch2" class="Str"("Text.BGColor"=w866) -> ()  [unwired: 2 in, 2 out]
                    n410 = property on="Acq status string ch1" class="Str"("Text.BGColor"=w872) -> ()  [unwired: 2 in, 2 out]
                    n411 = property on="Acq status string ch3" class="Str"("Text.BGColor"=w862) -> ()  [unwired: 2 in, 2 out]
                    n412 = property on="Acq status string ch4" class="Str"("Text.BGColor"=w858) -> ()  [unwired: 2 in, 2 out]
                  }
                  frame #3 {
                    w942 = cluster{u32, u32}[] [{16711680, 16711680}, {15400704, 15400704}, {16776722, 0}, {16776722, 0}]  # amarelo
                    w941 = cluster{u32, u32}[] [{16711680, 16711680}, {6618880, 6618880}, {16776722, 0}, {16776722, 0}]  # verde
                    # "Se ocupacao do disco maior que\n90%, barra em vermelho."
                    # "Atualiza status CANAL 1"
                    n413 = Unbundle By Name(w954) -> ("Frames done"=w951:u32, "connection"=→"Channel 1" →"setupCH1":bool, "conf runing"=w952:bool, "UsedDisk"=w936:u16, "operational"=w939:bool)
                    "Exposures Done ch1" <- w951
                    "Disk Storage ch1" <- w936
                    n414 = Number To Decimal String(number=w951) -> (decimal integer string=w949:string)  [unwired: 1 in]
                    n415 = Greater?(x=w936, y=u16 90) -> (0:w946:bool)
                    n416 = Select(t=u32 16711680, s=w946, f=u32 16860) -> (s? t:f=w944:u32)
                    n417 = Concatenate Strings("#Exposures Done ", w949) -> (w948:string)
                    n418 = Select(t=w941, s=w939, f=w942) -> (s? t:f=w940:cluster{u32, u32}[])
                    n419 = property on="setupCH1" class="Bool (strict)"("Blinking"=w952) -> ()  [unwired: 2 in, 2 out]
                    n420 = property on="Exposures Done ch1" class="Slide (strict)"("Caption.Text"=w948) -> ()  [unwired: 2 in, 2 out]
                    n421 = property on="Channel 1" class="Bool (strict)"("Colors [4]"=w940) -> ()  [unwired: 2 in, 2 out]
                    n422 = property on="Disk Storage ch1" class="Slide (strict)"("Fill Color"=w944) -> ()  [unwired: 2 in, 2 out]
                    n423 = Number To Decimal String(number=w936) -> (decimal integer string=w937:string)  [unwired: 1 in]
                    n424 = Concatenate Strings("Disk Storage ", w937, "%" ("string")) -> (w935:string)
                    n425 = property on="Disk Storage ch1" class="Slide (strict)"("Caption.Text"=w935) -> ()  [unwired: 2 in, 2 out]
                  }
                  frame #4 {
                    w963 = cluster{u32, u32}[] [{16711680, 16711680}, {15400704, 15400704}, {16776722, 0}, {16776722, 0}]  # amarelo
                    w962 = cluster{u32, u32}[] [{16711680, 16711680}, {6618880, 6618880}, {16776722, 0}, {16776722, 0}]  # verde
                    # "Se ocupacao do disco maior que\n90%, barra em vermelho."
                    # "Atualiza status CANAL 2"
                    n426 = Unbundle By Name(w975) -> ("Frames done"=w970:u32, "connection"=→"Channel 2" →"setupCH2":bool, "conf runing"=w973:bool, "UsedDisk"=w955:u16, "operational"=w960:bool)
                    "Exposures Done ch2" <- w970
                    "Disk Storage ch2" <- w955
                    n427 = Number To Decimal String(number=w970) -> (decimal integer string=w971:string)  [unwired: 1 in]
                    n428 = Greater?(x=w955, y=u16 90) -> (0:w967:bool)
                    n429 = Select(t=u32 16711680, s=w967, f=u32 16860) -> (s? t:f=w964:u32)
                    n430 = Concatenate Strings("#Exposures Done ", w971) -> (w969:string)
                    n431 = Select(t=w962, s=w960, f=w963) -> (s? t:f=w961:cluster{u32, u32}[])
                    n432 = property on="setupCH2" class="Bool (strict)"("Blinking"=w973) -> ()  [unwired: 2 in, 2 out]
                    n433 = property on="Disk Storage ch2" class="Slide (strict)"("Fill Color"=w964) -> ()  [unwired: 2 in, 2 out]
                    n434 = property on="Exposures Done ch2" class="Slide (strict)"("Caption.Text"=w969) -> ()  [unwired: 2 in, 2 out]
                    n435 = property on="Channel 2" class="Bool (strict)"("Colors [4]"=w961) -> ()  [unwired: 2 in, 2 out]
                    n436 = Number To Decimal String(number=w955) -> (decimal integer string=w958:string)  [unwired: 1 in]
                    n437 = Concatenate Strings("Disk Storage ", w958, "%" ("string")) -> (w956:string)
                    n438 = property on="Disk Storage ch2" class="Slide (strict)"("Caption.Text"=w956) -> ()  [unwired: 2 in, 2 out]
                  }
                  frame #5 {
                    w984 = cluster{u32, u32}[] [{16711680, 16711680}, {15400704, 15400704}, {16776722, 0}, {16776722, 0}]  # amarelo
                    w983 = cluster{u32, u32}[] [{16711680, 16711680}, {6618880, 6618880}, {16776722, 0}, {16776722, 0}]  # verde
                    # "Se ocupacao do disco maior que\n90%, barra em vermelho."
                    # "Atualiza status CANAL3"
                    n439 = Unbundle By Name(w996) -> ("Frames done"=w991:u32, "connection"=→"Channel 3" →"setupCH3":bool, "conf runing"=w995:bool, "UsedDisk"=w977:u16, "operational"=w982:bool)
                    "Exposures Done ch3" <- w991
                    "Disk Storage ch3" <- w977
                    n440 = Number To Decimal String(number=w991) -> (decimal integer string=w992:string)  [unwired: 1 in]
                    n441 = Greater?(x=w977, y=u16 90) -> (0:w988:bool)
                    n442 = Select(t=u32 16711680, s=w988, f=u32 16860) -> (s? t:f=w985:u32)
                    n443 = Concatenate Strings("#Exposures Done ", w992) -> (w990:string)
                    n444 = property on="setupCH3" class="Bool (strict)"("Blinking"=w995) -> ()  [unwired: 2 in, 2 out]
                    n445 = property on="Disk Storage ch3" class="Slide (strict)"("Fill Color"=w985) -> ()  [unwired: 2 in, 2 out]
                    n446 = Select(t=w983, s=w982, f=w984) -> (s? t:f=w981:cluster{u32, u32}[])
                    n447 = property on="Exposures Done ch3" class="Slide (strict)"("Caption.Text"=w990) -> ()  [unwired: 2 in, 2 out]
                    n448 = property on="Channel 3" class="Bool (strict)"("Colors [4]"=w981) -> ()  [unwired: 2 in, 2 out]
                    n449 = Number To Decimal String(number=w977) -> (decimal integer string=w979:string)  [unwired: 1 in]
                    n450 = Concatenate Strings("Disk Storage ", w979, "%" ("string")) -> (w976:string)
                    n451 = property on="Disk Storage ch3" class="Slide (strict)"("Caption.Text"=w976) -> ()  [unwired: 2 in, 2 out]
                  }
                  frame #6 {
                    w1005 = cluster{u32, u32}[] [{16711680, 16711680}, {15400704, 15400704}, {16776722, 0}, {16776722, 0}]  # amarelo
                    w1004 = cluster{u32, u32}[] [{16711680, 16711680}, {6618880, 6618880}, {16776722, 0}, {16776722, 0}]  # verde
                    # "Se ocupacao do disco maior que\n90%, barra em vermelho."
                    # "Atualiza status CANAL4"
                    n452 = Unbundle By Name(w1017) -> ("Frames done"=w1012:u32, "connection"=→"Channel 4" →"setupCH4":bool, "conf runing"=w1016:bool, "UsedDisk"=w998:u16, "operational"=w1002:bool)
                    "Exposures Done ch4" <- w1012
                    "Disk Storage ch4" <- w998
                    n453 = Number To Decimal String(number=w1012) -> (decimal integer string=w1013:string)  [unwired: 1 in]
                    n454 = Greater?(x=w998, y=u16 90) -> (0:w1009:bool)
                    n455 = Select(t=u32 16711680, s=w1009, f=u32 16860) -> (s? t:f=w1006:u32)
                    n456 = Concatenate Strings("#Exposures Done ", w1013) -> (w1011:string)
